vi "left.vi"(7 "Parâmetros Ini 2":T2={"Gyro Port"=0, "Sensor - Left"=3, "Sensor - Right"=2, "     Color \nSensor Port"=1, "Kp Front"=0.5, "Motor speed"=-15, "Distance to street"=0.0, "Motor speed turns"=16, "Kp Curvas"=0.3} {"Kp Front" format="%.3f"; "Color \nSensor Port" items=["Port 1", "Port 2", "Port 3", "Port 4"]; "Sensor - Right" items=["Port 1", "Port 2", "Port 3", "Port 4"]; "Sensor - Left" items=["Port 1", "Port 2", "Port 3", "Port 4"]; "Gyro Port" items=["Port 1", "Port 2", "Port 3", "Port 4"]}, 9 "NXT/EV3":T1) -> (0 "x = y?":bool, 1 "NXT/EV3 2":T1)   [LabVIEW 2016]
uses:
  <vilib>/NXT/Subs/LVHSConnector.ctl
  <vilib>/NXT/LegoClasses/BrickReference/BrickReference.lvclass
  parametros.ctl
  <vilib>/NXT/Block Support/NXT_InputPort.ctl
  <vilib>/NXT/Block Support/NXT_OutputPort.ctl
  <vilib>/NXT/Dual Mode Library/Sensors/EV3_Gyro_Angle.vi
  <vilib>/NXT/NXTIO Xnodes/NXTIONodeSubVIs/NXTMoveMotors.vi
  <vilib>/NXT/NXTIO Xnodes/NXTIONodeSubVIs/NXTStopMotors.vi
  <vilib>/NXT/NXTIO Xnodes/AddressXNode/NXTIOAddress.xnode
  <vilib>/NXT/NXTIO Xnodes/NXTIOXNode/NXTIO.xnode
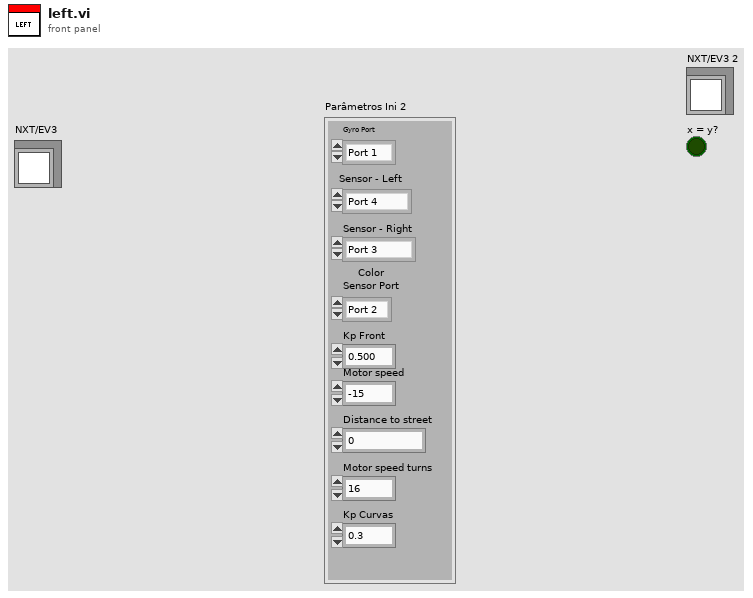
[diagram p1: front panel]
types:
  T1 = typedef "LVHSConnector.ctl" = refnum<class "BrickReference.lvclass">
  T2 = typedef "parametros.ctl" = cluster{"Gyro Port":T3, "Sensor - Left":T3, "Sensor - Right":T3, "     Color \nSensor Port":T3, "Kp Front":dbl, "Motor speed":i32, "Distance to street":dbl, "Motor speed turns":i32, "Kp Curvas":dbl}
  T3 = typedef "NXT_InputPort.ctl" = u32
  T4 = typedef "NXT_OutputPort.ctl" = u8
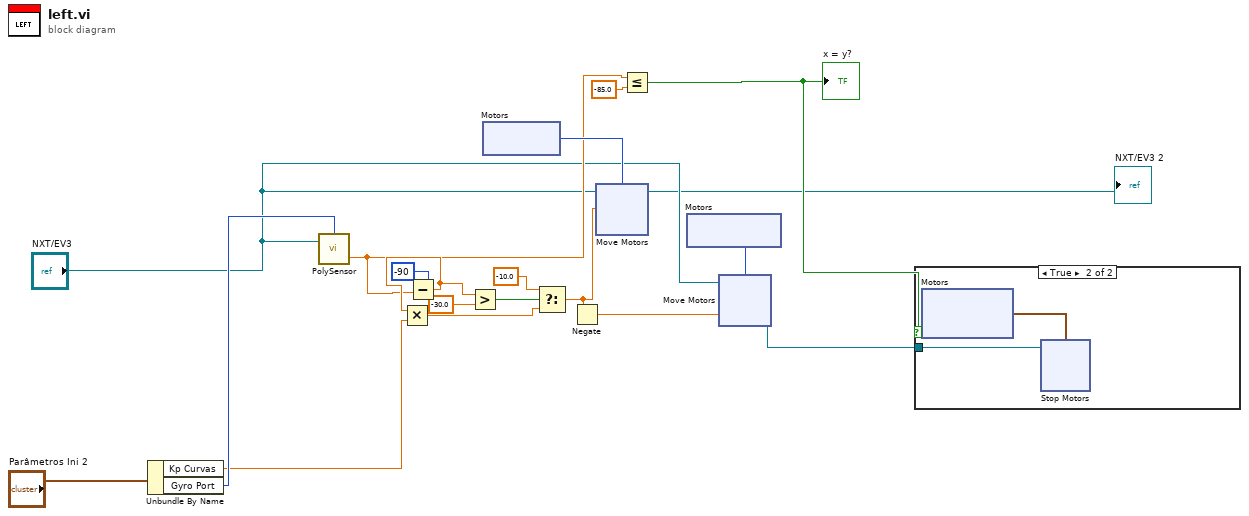
[diagram p0: block diagram]
diagram:
  n1 = Unbundle By Name("Parâmetros Ini 2") -> ("Kp Curvas"=w17:dbl, "Gyro Port"=w19:T3)
  n2 = call-poly <vilib>:"PolySensor.vi"("NXT/EV3"="NXT/EV3", "Port (Port 1)"=w19) -> ("Degrees"=w7:sgl)  [unwired: 1 in, 1 out]
  n3 = Subtract(x=-90, y=w7) -> (x-y=w10:sgl)
  n4 = Multiply(x=w10, y=w17) -> (x*y=w8:dbl)
  n5 = Greater?(x=w10, y=sgl -30.0) -> (0:w14:bool)
  n6 = xnode "Motors"() -> ("Motor"=w13:T4)
  n7 = Select(t=sgl -10.0, s=w14, f=w8) -> (s? t:f=w5:dbl)
  n8 = Negate(x=w5) -> (-x=w6:dbl)
  n9 = xnode "Move Motors"("Power/Speed 1"=w5, "Motors"=w13, "NXT/EV3"="NXT/EV3") -> ("NXT/EV3"=→"NXT/EV3 2":T1)
  n10 = Less Or Equal?(x=w7, y=sgl -85.0) -> (x <= y?=w3:bool)
  "x = y?" <- w3
  n11 = xnode "Motors"() -> ("Motor"=w12:T4)
  n12 = xnode "Move Motors"("Power/Speed 1"=w6, "Motors"=w12, "NXT/EV3"="NXT/EV3") -> ("NXT/EV3"=w2:T1)
  n13 = case shown="True" w3 {
    tunnel: w2 -> [_ w20]
    frame False {
    }
    frame True {
      n14 = xnode "Motors"() -> ("Motor"=w21:cluster{"Port":T4, "Port":T4})
      n15 = xnode "Stop Motors"("Motors"=w21, "NXT/EV3"=w20) -> ()  [unwired: 1 out]
    }
  }
